vi "SignUp(SubVI).vi"() -> ()   [LabVIEW 2013]
uses:
  <vilib>/addons/database/Connection.llb/DB Tools Open Connec (String).vi
  FYP_LabviewGlobal(SubVI).vi
  <vilib>/addons/database/_DB Variant To Data/Database Variant To Data.xnode
  <vilib>/addons/database/NI_Database_API.lvlib
panel:
  out "Nameblank?":string="REQUIRED"
  out "Confirm Passwordblank?":string="ERQUIRED"
  out "PasswordBlnk?":string="REQUIRED"
  out "Confirm AdminNoBlank?":string="REQUIRED"
  out "Admin no blank?":string="REQUIRED"
  out "ADMINNO.EXISTS?":bool
  out "AdminNo.Accepted?":string
  out "PasswordMismatching":string="PASSWORD MISMATCHING"
  out "AdminNoMismatching":string="ADMIN NO MISMATCHING"
  in  "Submit":bool
  in  "Confirm password:":string
  in  "Password:":string
  in  "Confirm Admin no.:":string
  in  "Admin no.:":string
  in  "Name:":string
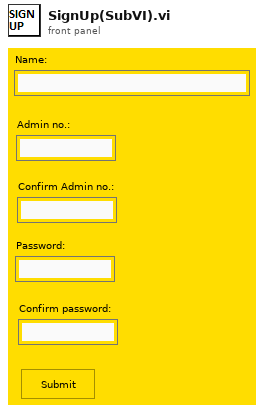
[diagram p1: front panel]
types:
  T1 = typedef "NI_Database_API.lvlib/Conn ObjectReference.ctl" = refnum<k1>
  T2 = cluster{"Name:":string, string, "Password:":string}
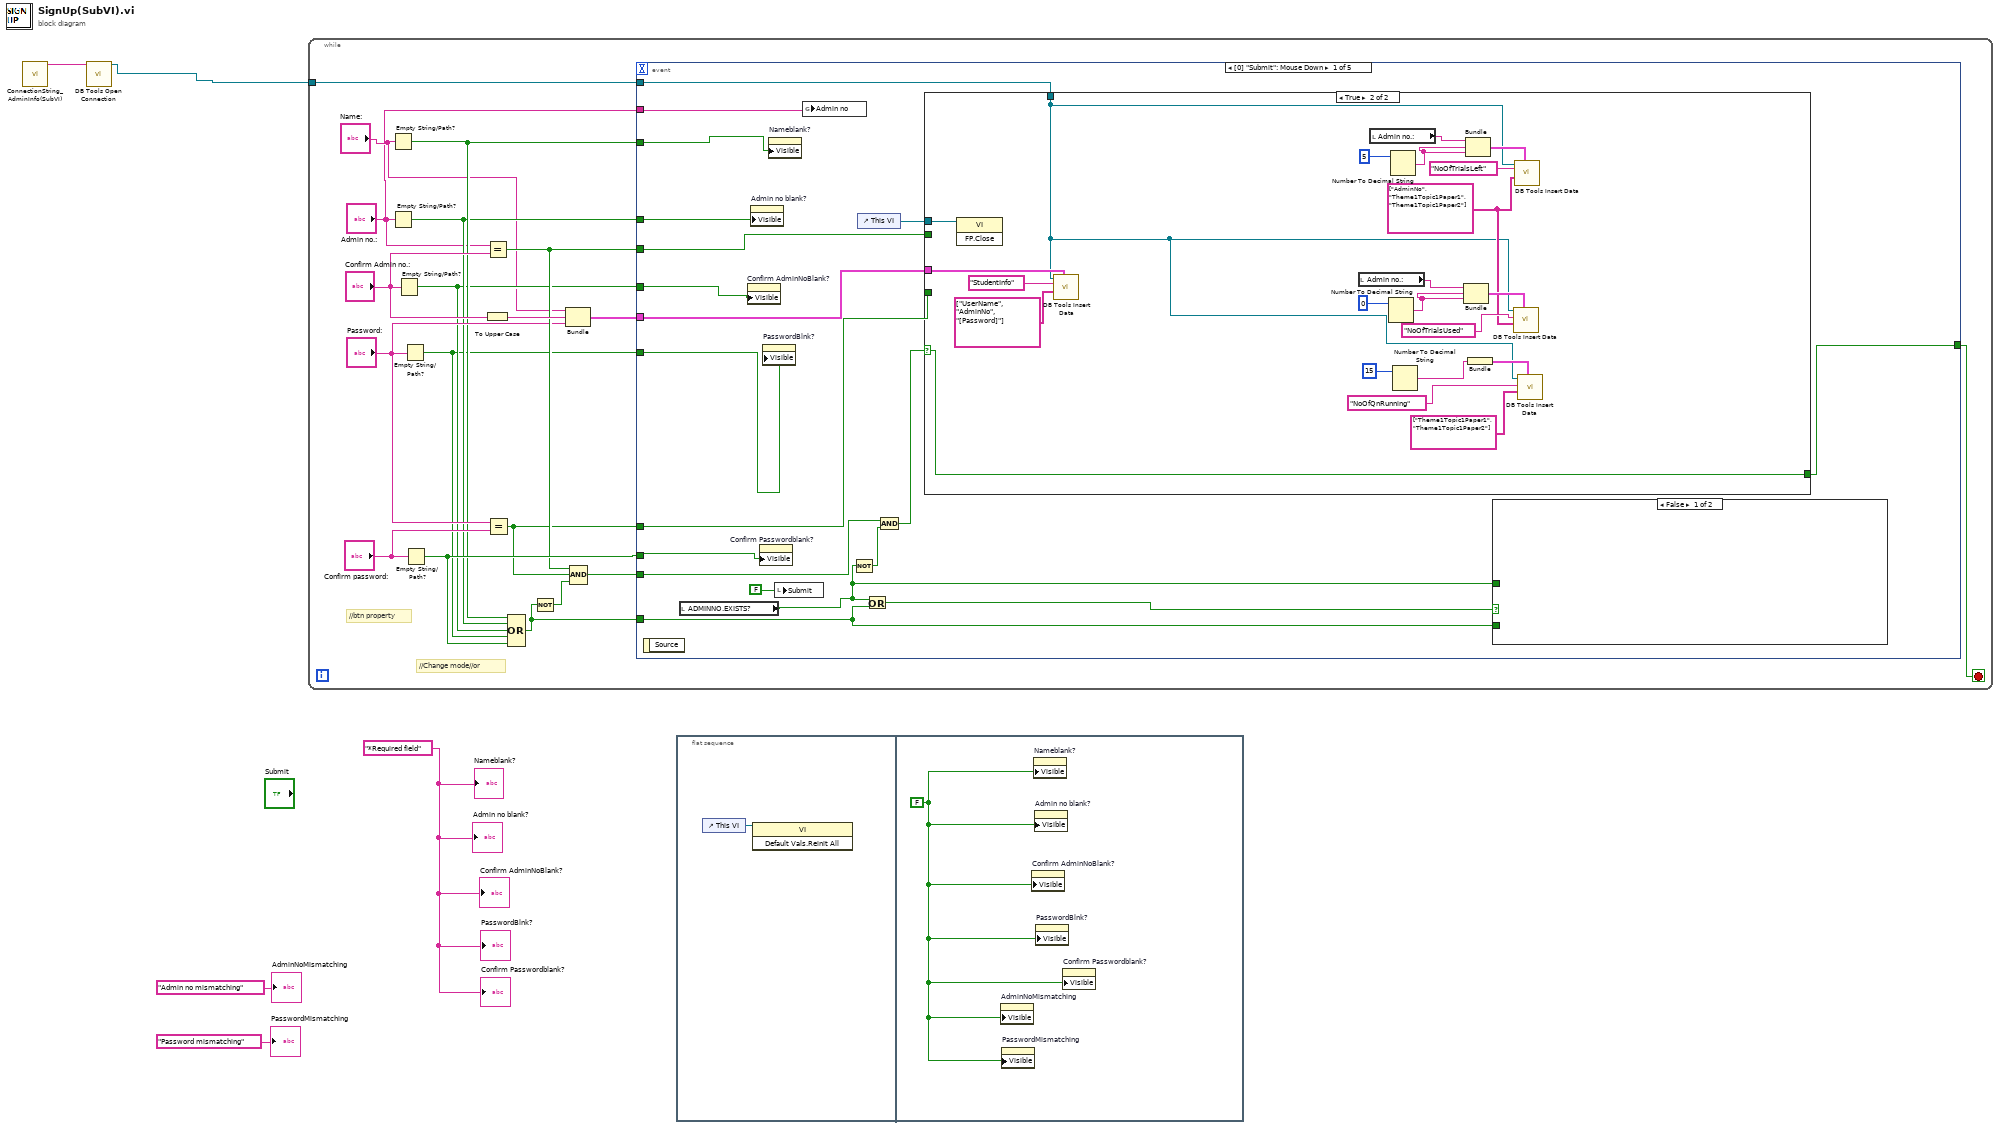
[diagram p0: block diagram]
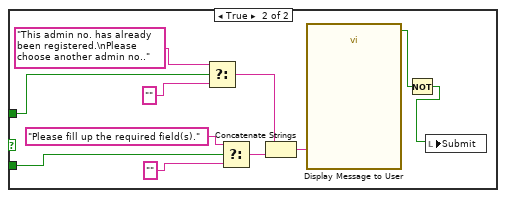
[diagram p2: hidden frame]
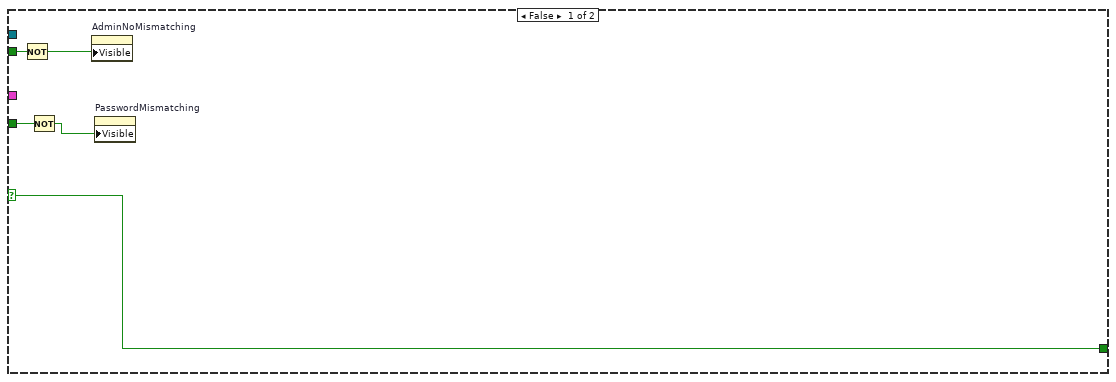
[diagram p3: hidden frame]
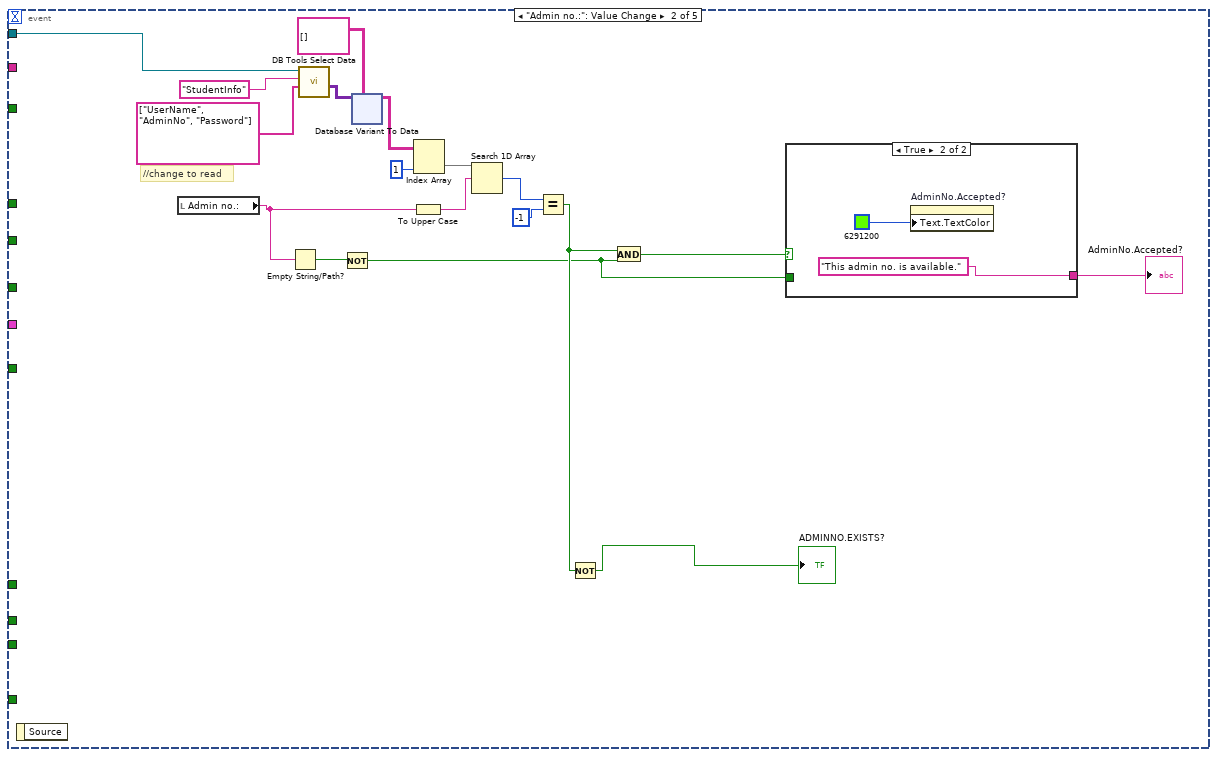
[diagram p4: hidden frame]
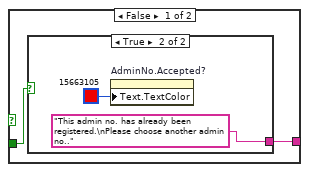
[diagram p5: hidden frame]
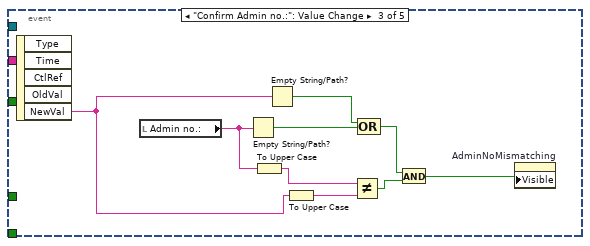
[diagram p7: hidden frame]
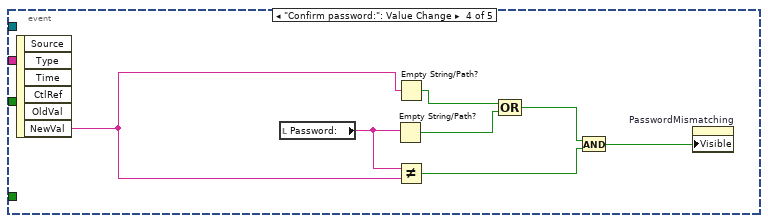
[diagram p8: hidden frame]
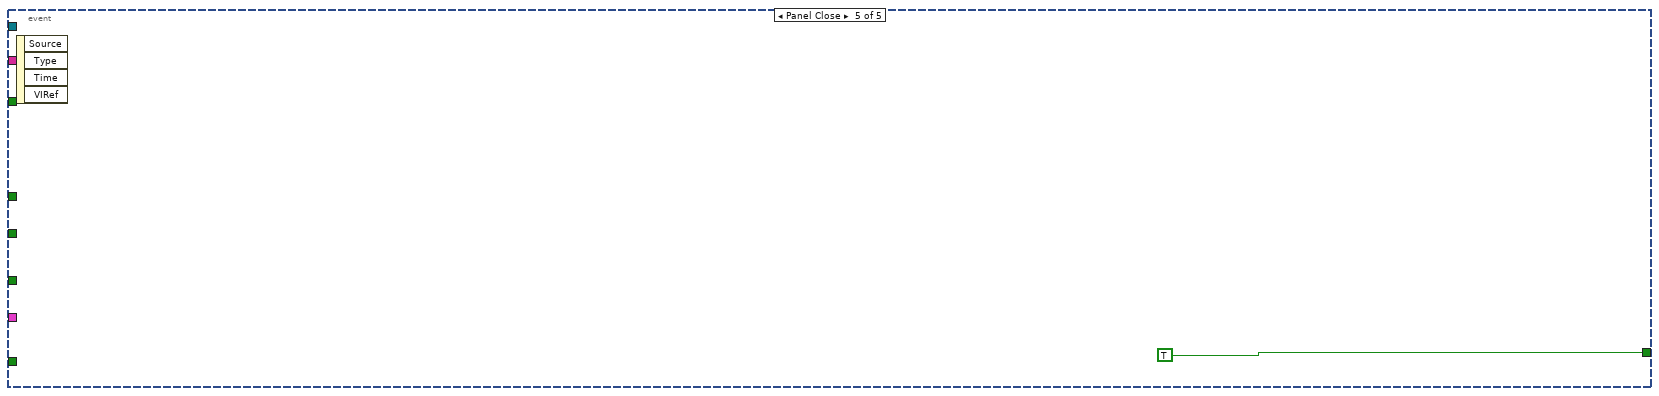
[diagram p9: hidden frame]
diagram:
  w3 = "*Required field"
  n1 = call "ConnectionString_AdminInfo(SubVI).vi"() -> ("ConnectionString"=w2:string)  [unwired: 11 in]
  n2 = call-poly <vilib>:"DB Tools Open Connection.vi"("connection information"=w2) -> ("connection reference"=w1:T1)  [unwired: 7 in, 1 out]
  n3 = while {
    tunnel: w1 -> [w16]
    stop <- w13 stop-if-true
    # "//btn property"
    # "//Change mode//or"
    n4 = Empty String/Path?(string/path="Name:") -> (empty?=w11:bool)
    n5 = Empty String/Path?(string/path="Admin no.:") -> (empty?=w10:bool)
    n6 = Empty String/Path?(string/path="Confirm Admin no.:") -> (empty?=w9:bool)
    n7 = Empty String/Path?(string/path="Password:") -> (empty?=w8:bool)
    n8 = Empty String/Path?(string/path="Confirm password:") -> (empty?=w20:bool)
    n9 = To Upper Case(1:"Confirm Admin no.:") -> (0:w22:string)
    n10 = Equal?(x="Admin no.:", y="Confirm Admin no.:") -> (x = y?=w15:bool)
    n11 = Equal?(x="Password:", y="Confirm password:") -> (x = y?=w14:bool)
    n12 = Compound Arithmetic op=OR(w11, w10, w9, w8, w20) -> (w18:bool)
    n13 = Not(x=w18) -> (.not. x?=w21:bool)
    n14 = Bundle("Name:"="Name:", w22, "Password:"="Password:") -> (w17:T2)  [unwired: 1 in]
    n15 = Compound Arithmetic op=AND(w15, w14, w21) -> (w19:bool)
    n16 = event shown="[0] \"Submit\": Mouse Down" {
      selector: _ -> [_ _ _ _ _]
      dyn-events: _ -> [_ _ _ _ _]
      timeout: _ -> [_ _ _ _ _]
      tunnel: w11 -> [w26 _ _ _ _]
      tunnel: w10 -> [w27 _ _ _ _]
      tunnel: w9 -> [w28 _ _ _ _]
      tunnel: w8 -> [w29 _ _ _ _]
      tunnel: w20 -> [w30 _ _ _ _]
      tunnel: w19 -> [w37 _ _ _ _]
      tunnel: w18 -> [w33 _ _ _ _]
      tunnel: w17 -> [w40 _ _ _ _]
      tunnel: w16 -> [w43 w84 _ _ _]
      tunnel: w15 -> [w41 _ _ _ _]
      tunnel: w14 -> [w39 _ _ _ _]
      tunnel: [w35 _ _ _ TRUE] -> w13
      tunnel: "Admin no.:" -> [w25 _ _ _ _]
      event "Submit": Mouse Down {
        n17 = event-data() -> ()  [unwired: 1 in, 1 out]
        n18 = local read "ADMINNO.EXISTS?"() -> (w31:bool)
        n19 = property on="Confirm AdminNoBlank?" class="Str"("Visible"=w28) -> ()  [unwired: 2 in, 2 out]
        n20 = property on="Admin no blank?" class="Str"("Visible"=w27) -> ()  [unwired: 2 in, 2 out]
        n21 = property on="Confirm Passwordblank?" class="Str"("Visible"=w30) -> ()  [unwired: 2 in, 2 out]
        n22 = property on="PasswordBlnk?" class="Str"("Visible"=w29) -> ()  [unwired: 2 in, 2 out]
        n23 = property on="Nameblank?" class="Str"("Visible"=w26) -> ()  [unwired: 2 in, 2 out]
        n24 = local write "Submit"(FALSE) -> ()
        n25 = global write "FYP_LabviewGlobal(SubVI).vi" "Admin no"(w25) -> ()
        n26 = Not(x=w31) -> (.not. x?=w34:bool)
        n27 = control-ref of="This VI"() -> (w42:refnum<vi>)
        n28 = Or(x=w31, y=w33) -> (x .or. y?=w32:bool)
        n29 = And(x=w37, y=w34) -> (x .and. y?=w38:bool)
        n30 = case shown="True" w38 {
          selector: w38 -> [w55 w81]
          tunnel: w43 -> [_ w61]
          tunnel: w42 -> [_ w80]
          tunnel: w41 -> [w59 _]
          tunnel: w40 -> [_ w78]
          tunnel: w39 -> [w58 _]
          tunnel: [w55 w81] -> w35
          frame False {
            n31 = Not(x=w59) -> (.not. x?=w56:bool)
            n32 = Not(x=w58) -> (.not. x?=w57:bool)
            n33 = property on="AdminNoMismatching" class="Str"("Visible"=w56) -> ()  [unwired: 2 in, 2 out]
            n34 = property on="PasswordMismatching" class="Str"("Visible"=w57) -> ()  [unwired: 2 in, 2 out]
          }
          frame True {
            w66 = string[] ["AdminNo", "Theme1Topic1Paper1", "Theme1Topic1Paper2"] ("columns")
            n35 = invoke class="VI" method="FP.Close"(reference=w80) -> ()  [unwired: 2 in, 3 out]
            n36 = call <vilib>:"DB Tools Insert Data.vi"("data"=w78, "columns"=string[] ["UserName", "AdminNo", "[Password]"], "table"="StudentInfo", "connection reference"=w61) -> ()  [unwired: 6 in, 2 out]
            n37 = local read "Admin no.:"() -> (w67:string)
            n38 = local read "Admin no.:"() -> (w75:string)
            n39 = Number To Decimal String(number=0) -> (decimal integer string=w69:string)  [unwired: 1 in]
            n40 = Number To Decimal String(number=5) -> (decimal integer string=w73:string)  [unwired: 1 in]
            n41 = Number To Decimal String(number=15) -> (decimal integer string=w63:string)  [unwired: 1 in]
            n42 = Bundle("Admin no.:"=w67, w69, w69) -> (w70:cluster{"Admin no.:":string, string, string})  [unwired: 1 in]
            n43 = Bundle("Admin no.:"=w75, w73, w73) -> (w74:cluster{"Admin no.:":string, string, string})  [unwired: 1 in]
            n44 = Bundle(w63) -> (w64:cluster{string})  [unwired: 1 in]
            n45 = call <vilib>:"DB Tools Insert Data.vi"("data"=w70, "columns"=w66, "table"="NoOfTrialsUsed", "connection reference"=w61) -> ()  [unwired: 6 in, 2 out]
            n46 = call <vilib>:"DB Tools Insert Data.vi"("data"=w74, "columns"=w66, "table"="NoOfTrialsLeft", "connection reference"=w61) -> ()  [unwired: 6 in, 2 out]
            n47 = call <vilib>:"DB Tools Insert Data.vi"("data"=w64, "columns"=string[] ["Theme1Topic1Paper1", "Theme1Topic1Paper2"], "table"="NoOfQnRunning", "connection reference"=w61) -> ()  [unwired: 6 in, 2 out]
          }
        }
        n48 = case shown="False" w32 {
          tunnel: w33 -> [_ w49]
          tunnel: w31 -> [_ w54]
          frame False {
          }
          frame True {
            n49 = Select(t="This admin no. has already been registered.\nPlease choose another admin no..", s=w54, f="") -> (s? t:f=w48:string)
            n50 = Select(t="Please fill up the required field(s).", s=w49, f="") -> (s? t:f=w47:string)
            n51 = Concatenate Strings(w48, w47) -> (w44:string)
            n52 = call "Display Message to User"("Message"=w44) -> ("OK"=w46:bool)  [unwired: 9 in, 1 out]
            n53 = Not(x=w46) -> (.not. x?=w45:bool)
            n54 = local write "Submit"(w45) -> ()
          }
        }
      }
      event "Admin no.:": Value Change {
        # "//change to read"
        n55 = event-data() -> ()  [unwired: 1 in, 1 out]
        n56 = local read "Admin no.:"() -> (w90:string)
        n57 = Empty String/Path?(string/path=w90) -> (empty?=w89:bool)
        n58 = call <vilib>:"DB Tools Select Data.vi"("columns"=string[] ["UserName", "AdminNo", "Password"], "table"="StudentInfo", "connection reference"=w84) -> ("data"=w98:variant[][])  [unwired: 3 in, 2 out]
        n59 = Not(x=w89) -> (.not. x?=w86:bool)
        n60 = xnode "Database Variant To Data"("database variant"=w98, "type"=string[][] []) -> ("data"=w96:string[][])  [unwired: 1 in, 1 out]
        n61 = To Upper Case(1:w90) -> (0:w93:string)
        n62 = Index Array(array=w96, index (col)=1) -> (element=w94:string[])  [unwired: 1 in]
        n63 = Search 1D Array(1D array=w94, element=w93) -> (index of element=w92:i32)  [unwired: 1 in]
        n64 = Equal?(x=w92, y=-1) -> (x = y?=w88:bool)
        n65 = Not(x=w88) -> (.not. x?=→"ADMINNO.EXISTS?":bool)
        n66 = And(x=w88, y=w86) -> (x .and. y?=w87:bool)
        n67 = case shown="True" w87 {
          tunnel: w86 -> [w100 _]
          tunnel: [w101 "This admin no. is available."] -> w85
          frame False {
            n68 = case shown="True" w100 {
              tunnel: [_ "This admin no. has already been registered.\nPlease choose another admin no.."] -> w101
              frame False {
              }
              frame True {
                n69 = property on="AdminNo.Accepted?" class="Str"("Text.TextColor"=u32 15663105) -> ()  [unwired: 2 in, 2 out]
              }
            }
          }
          frame True {
            n70 = property on="AdminNo.Accepted?" class="Str"("Text.TextColor"=u32 6291200) -> ()  [unwired: 2 in, 2 out]
          }
        }
        "AdminNo.Accepted?" <- w85
      }
      event "Confirm Admin no.:": Value Change {
        n71 = event-data() -> ("NewVal"=w158:string)  [unwired: 1 in, 4 out]
        n72 = local read "Admin no.:"() -> (w157:string)
        n73 = Empty String/Path?(string/path=w157) -> (empty?=w155:bool)
        n74 = To Upper Case(1:w157) -> (0:w154:string)
        n75 = Empty String/Path?(string/path=w158) -> (empty?=w156:bool)
        n76 = To Upper Case(1:w158) -> (0:w153:string)
        n77 = Not Equal?(x=w154, y=w153) -> (x != y?=w152:bool)
        n78 = Compound Arithmetic op=OR(w156, w155) -> (w151:bool)
        n79 = And(x=w151, y=w152) -> (x .and. y?=w150:bool)
        n80 = property on="AdminNoMismatching" class="Str"("Visible"=w150) -> ()  [unwired: 2 in, 2 out]
      }
      event "Confirm password:": Value Change {
        n81 = event-data() -> ("NewVal"=w165:string)  [unwired: 1 in, 5 out]
        n82 = local read "Password:"() -> (w164:string)
        n83 = Empty String/Path?(string/path=w164) -> (empty?=w162:bool)
        n84 = Empty String/Path?(string/path=w165) -> (empty?=w163:bool)
        n85 = Not Equal?(x=w164, y=w165) -> (x != y?=w160:bool)
        n86 = Compound Arithmetic op=OR(w163, w162) -> (w161:bool)
        n87 = And(x=w161, y=w160) -> (x .and. y?=w159:bool)
        n88 = property on="PasswordMismatching" class="Str"("Visible"=w159) -> ()  [unwired: 2 in, 2 out]
      }
      event Panel Close {
        n89 = event-data() -> ()  [unwired: 1 in, 4 out]
      }
    }
  }
  n90 = flat-sequence {
    frame #0 {
      n91 = control-ref of="This VI"() -> (w167:refnum<vi>)
      n92 = invoke class="VI" method="Default Vals.Reinit All"(reference=w167) -> ()  [unwired: 2 in, 3 out]
    }
    frame #1 {
      w168 = FALSE
      n93 = property on="AdminNoMismatching" class="Str"("Visible"=w168) -> ()  [unwired: 2 in, 2 out]
      n94 = property on="PasswordMismatching" class="Str"("Visible"=w168) -> ()  [unwired: 2 in, 2 out]
      n95 = property on="Confirm AdminNoBlank?" class="Str"("Visible"=w168) -> ()  [unwired: 2 in, 2 out]
      n96 = property on="Nameblank?" class="Str"("Visible"=w168) -> ()  [unwired: 2 in, 2 out]
      n97 = property on="Admin no blank?" class="Str"("Visible"=w168) -> ()  [unwired: 2 in, 2 out]
      n98 = property on="PasswordBlnk?" class="Str"("Visible"=w168) -> ()  [unwired: 2 in, 2 out]
      n99 = property on="Confirm Passwordblank?" class="Str"("Visible"=w168) -> ()  [unwired: 2 in, 2 out]
    }
  }
  "AdminNoMismatching" <- "Admin no mismatching" ("AdminNoMismatching")
  "PasswordMismatching" <- "Password mismatching" ("PasswordMismatching")
  "Admin no blank?" <- w3
  "Confirm AdminNoBlank?" <- w3
  "PasswordBlnk?" <- w3
  "Confirm Passwordblank?" <- w3
  "Nameblank?" <- w3
